vi "Async-Message with User Event.vi"() -> ()   [LabVIEW 2020, in "TCPRouter ClientAPI Examples.lvlib"]
uses:
  _addons/TCP-Router/ClientAPI/Def-TCP-Router Async-Resp Data.ctl
  84a30447-af23-4955-814f-601ed374970b.vi
  b3b63605-1016-4be4-a788-12e3256b011c.vi
  TCPRouter ClientAPI Examples.lvlib
  _addons/TCP-Router/ClientAPI/TcpRouter-Client.lvclass
panel:
  out "element":T1[](array[typedef])
  out "current time":timestamp
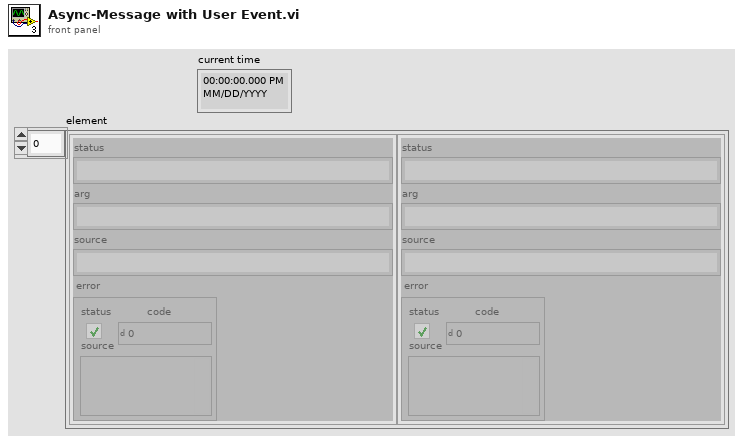
[diagram p1: front panel]
types:
  T1 = typedef "CSM-TCP-Router.lvlib/TcpRouter-Client.lvclass/Def-TCP-Router Async-Resp Data.ctl" = cluster{"status":string, "arg":string, "source":string, "error":errorcluster}
  T2 = cluster{"IP Address":string, "Port":u16, "ConnectTMO":i32}
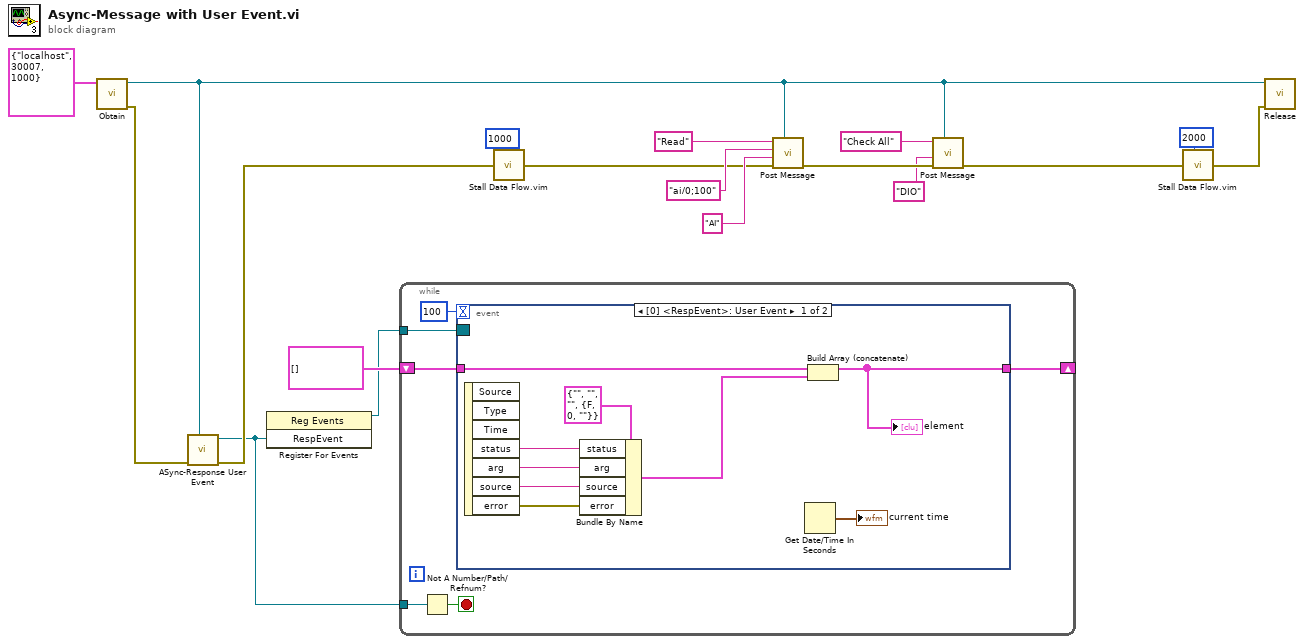
[diagram p0: block diagram]
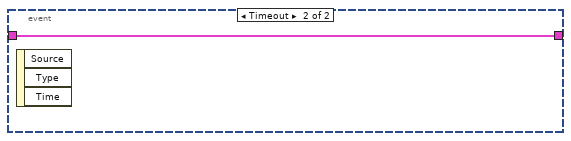
[diagram p2: hidden frame]
diagram:
  n1 = call "Obtain.vi"("Connection"=T2 {"IP Address"="localhost", "Port"=30007, "ConnectTMO"=1000}) -> ("error out"=w15:errorcluster, "TcpRouter-Client out"=w6:refnum<class "TcpRouter-Client.lvclass">)  [unwired: 9 in]
  n2 = call "ASync-Response User Event.vi"("TcpRouter-Client in"=w6, "error in (no error)"=w15) -> ("error out"=w7:errorcluster, "RespEvent"=w3:refnum<user-event>)  [unwired: 8 in]
  n3 = register-events(w3) -> (reference out=w4:refnum<event-registration>)  [unwired: 2 in, 1 out]
  n4 = while {
    shift-right: [w23] -> _
    shift-left: T1[] [] ("element") -> [w24]
    tunnel: w4 -> [w22]
    tunnel: w3 -> [w19]
    stop <- w20 stop-if-true
    n5 = Not A Number/Path/Refnum?(number/path/refnum=w19) -> (NaN/Path/Refnum?=w20:bool)
    n6 = event shown="[0] <RespEvent>: User Event" {
      selector: w22 -> [_ _]
      dyn-events: _ -> [_ _]
      timeout: 100 -> [_ _]
      tunnel: w24 -> [w32 w34]
      tunnel: [w31 w34] -> w23
      event User Event {
        n7 = event-data() -> ("status"=w29:string, "arg"=w28:string, "source"=w27:string, "error"=w26:errorcluster)  [unwired: 1 in, 3 out]
        n8 = Bundle By Name(cluster=T1 {"status"="", "arg"="", "source"="", "error"={"status"=FALSE, "code"=0, "source"=""}} ("element"), "status"=w29, "arg"=w28, "source"=w27, "error"=w26) -> (w25:T1)
        n9 = Get Date/Time In Seconds() -> (seconds since 1Jan1904=→"current time":timestamp)
        n10 = Build Array (concatenate)(w32, w25) -> (w31:T1[])
        "element" <- w31
      }
      event Timeout {
        n11 = event-data() -> ()  [unwired: 1 in, 3 out]
      }
    }
  }
  n12 = call "Stall Data Flow.vim"("value in"=w7, "milliseconds to wait"=u32 1000) -> ("value out"=w2:errorcluster)  [unwired: 1 out]
  n13 = call "Post Message.vi"("TcpRouter-Client in"=w6, "error in (no error)"=w2, "Target Module"="AI", "Arguments (\"\")"="ai/0;100" ("State"), "State"="Read") -> ("error out"=w11:errorcluster)  [unwired: 6 in]
  n14 = call "Post Message.vi"("TcpRouter-Client in"=w6, "error in (no error)"=w11, "Target Module"="DIO", "State"="Check All") -> ("error out"=w8:errorcluster)  [unwired: 7 in]
  n15 = call "Stall Data Flow.vim"("value in"=w8, "milliseconds to wait"=u32 2000) -> ("value out"=w17:errorcluster)  [unwired: 1 out]
  n16 = call "Release.vi"("error in (no error)"=w17, "TcpRouter-Client in"=w6) -> ()  [unwired: 9 in, 1 out]
